vi "tcp_connect.vi"(4 "Port":u16=5025, 6 "IP":string="192.168.2.29", 7 "button_tcp_connect":bool, 8 "error_in":errorcluster, 9 "tcp_connected_in":bool, 11 "connection_id_in":refnum<k5>) -> (0 "error out":errorcluster, 1 "tcp_connected_out":bool, 2 "new_connection":bool, 3 "connection_id_out":refnum<k5>)   [LabVIEW 2025]
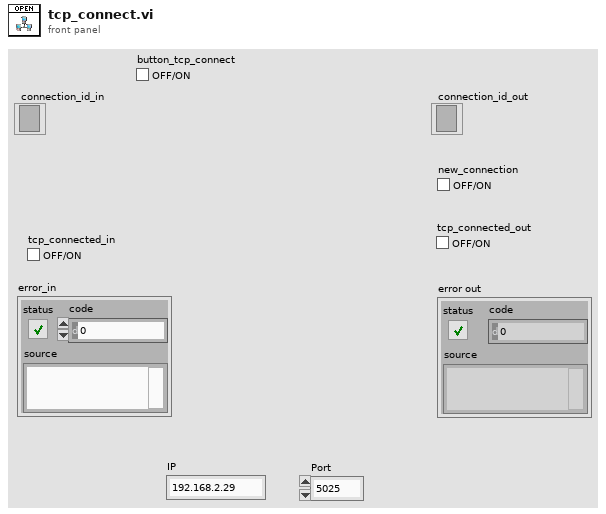
[diagram p1: front panel]
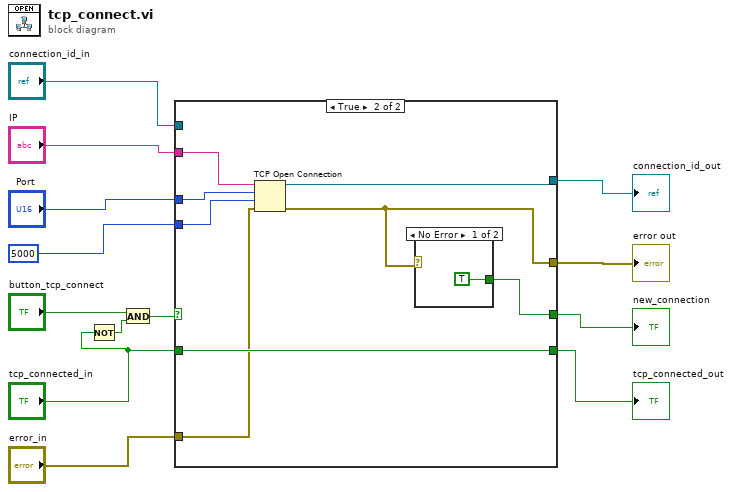
[diagram p0: block diagram]
diagram:
  n1 = Not(x="tcp_connected_in") -> (.not. x?=w11:bool)
  n2 = And(x="button_tcp_connect", y=w11) -> (x .and. y?=w13:bool)
  n3 = case shown="True" w13 {
    tunnel: 5000 ("timeout ms (60000)") -> [_ w23]
    tunnel: "Port" -> [_ w22]
    tunnel: "IP" -> [_ w21]
    tunnel: [_ w19] -> w7
    tunnel: [_ w18] -> w6
    tunnel: [w15 w17] -> w5
    tunnel: "tcp_connected_in" -> [w15 w17]
    tunnel: [w14 w20] -> w3
    tunnel: "error_in" -> [_ w16]
    tunnel: "connection_id_in" -> [w14 _]
    frame False {
    }
    frame True {
      n4 = TCP Open Connection(address=w21, remote port or service name=w22, timeout ms (60000)=w23, error in (no error)=w16) -> (connection ID=w20:refnum<k5>, error out=w19:errorcluster)  [unwired: 1 in]
      n5 = case shown="No Error" w19 {
        tunnel: [TRUE ("tcp_connected_in") _] -> w18
        frame No Error {
        }
        frame Error {
        }
      }
    }
  }
  "error out" <- w7
  "new_connection" <- w6
  "tcp_connected_out" <- w5
  "connection_id_out" <- w3
